vi "dice_vi.vi"() -> ()   [LabVIEW 2020]
panel:
  out "Dice":u16(ring)
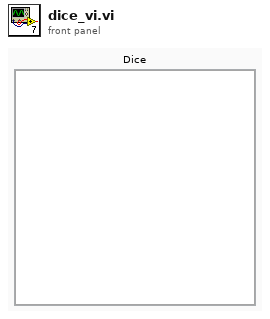
[diagram p1: front panel]
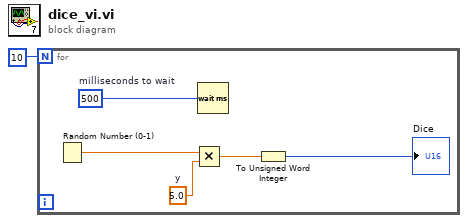
[diagram p0: block diagram]
diagram:
  n1 = for {
    N: 10 -> [_]
    w2 = u32 500  # milliseconds to wait
    w5 = 5.0  # y
    n2 = Random Number (0-1)() -> (number: 0 to 1=w6:dbl)
    n3 = Multiply(x=w6, y=w5) -> (x*y=w4:dbl)
    n4 = Wait (ms)(milliseconds to wait=w2) -> ()  [unwired: 1 out]
    n5 = To Unsigned Word Integer(number=w4) -> (unsigned 16bit integer=→"Dice":u16)
  }
